vi "New Line from Data.vi"(0 "Mode":string, 1 "DAQ A":dbl, 2 "Setting":dbl, 3 "DAQ R":dbl, 4 "BK V":dbl, 5 "Universal Time Stamp":dbl, 6 "DateTime Stamp":timestamp, 7 "BK I":dbl, 8 "RunName":string, 9 "BK R":dbl, 10 "Delimiter Character":string, 11 "BK P":dbl, 13 "DAQ T":dbl) -> (14 "String":string)   [LabVIEW 2010]
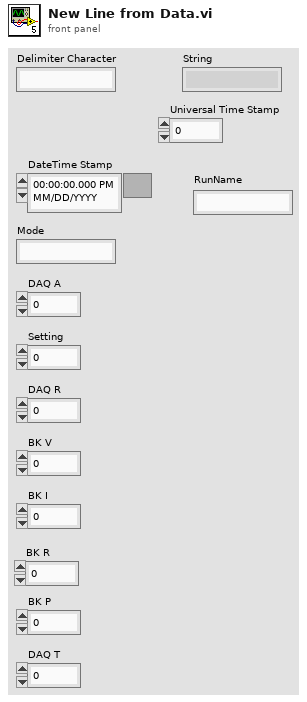
[diagram p1: front panel]
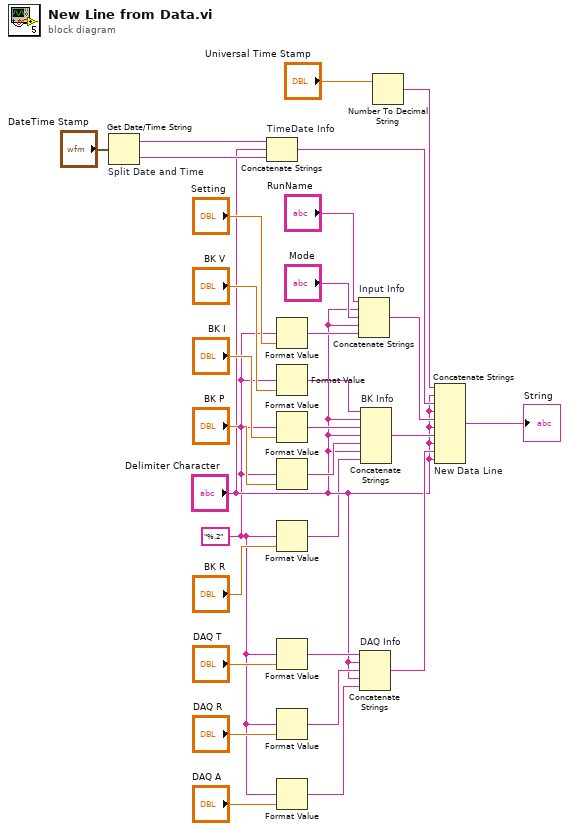
[diagram p0: block diagram]
diagram:
  w2 = "%.2"
  n1 = Get Date/Time String "Split Date and Time"(seconds (now)="DateTime Stamp") -> (date string=w15:string, time string=w16:string)  [unwired: 2 in]
  n2 = Concatenate Strings "TimeDate Info"(w15, "Delimiter Character", w16) -> (w6:string)
  n3 = Format Value(format string=w2, value (0)="Setting") -> (output string=w30:string)  [unwired: 1 in]
  n4 = Format Value(format string=w2, value (0)="BK V") -> (output string=w26:string)  [unwired: 1 in]
  n5 = Format Value(format string=w2, value (0)="BK I") -> (output string=w27:string)  [unwired: 1 in]
  n6 = Format Value(format string=w2, value (0)="BK P") -> (output string=w5:string)  [unwired: 1 in]
  n7 = Format Value(format string=w2, value (0)="BK R") -> (output string=w1:string)  [unwired: 1 in]
  n8 = Format Value(format string=w2, value (0)="DAQ T") -> (output string=w23:string)  [unwired: 1 in]
  n9 = Format Value(format string=w2, value (0)="DAQ R") -> (output string=w24:string)  [unwired: 1 in]
  n10 = Format Value(format string=w2, value (0)="DAQ A") -> (output string=w25:string)  [unwired: 1 in]
  n11 = Concatenate Strings "Input Info"("RunName", "Delimiter Character", "Mode", "Delimiter Character", w30) -> (w11:string)
  n12 = Concatenate Strings "DAQ Info"(w23, "Delimiter Character", w24, "Delimiter Character", w25) -> (w13:string)
  n13 = Concatenate Strings "BK Info"(w26, "Delimiter Character", w27, "Delimiter Character", w5, "Delimiter Character", w1) -> (w12:string)
  n14 = Number To Decimal String(number="Universal Time Stamp") -> (decimal integer string=w7:string)  [unwired: 1 in]
  n15 = Concatenate Strings "New Data Line"(w7, "Delimiter Character", w6, "Delimiter Character", w11, "Delimiter Character", w12, "Delimiter Character", w13, "Delimiter Character") -> (→"String":string)
